vi "Frame Wall Set.vi"(8 "error in (no error)":errorcluster, 9 "Wall Stiffness (N/m)":dbl=0.2 format="%#.1f", 10 "Restrict to Frame":bool=TRUE) -> (0 "error out":errorcluster)   [LabVIEW 2023, in "Haptic Prog Interface.lvlib"]
doc: "Restricts the haptic pen xy movement to a square canvas, and coerces all xy values to be within thie canvas.\n\n<b>Restrict to Frame:</b> Accepts a boolean, where a true value enables the frame wall.\n\n<b>Wall Stiffness:</b> Accepts a double, and changes the value k in F = k x, effectively changing the hardness of the wall.."
uses:
  Haptic Prog Interface.lvlib
  Haptic-Programming-Interface/src/x64/Debug/Haptic Programming Interface.dll
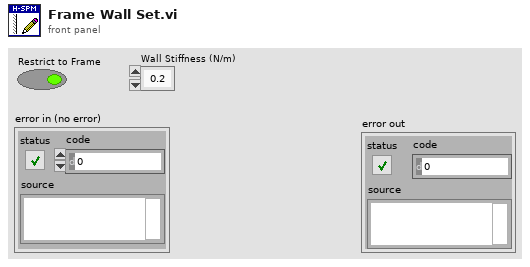
[diagram p1: front panel]
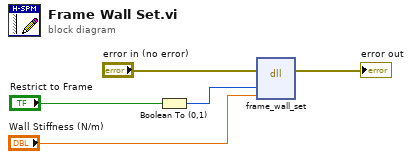
[diagram p0: block diagram]
diagram:
  n1 = Boolean To (0,1)(Boolean="Restrict to Frame") -> (0, 1=w3:i16)
  n2 = dll-call lib="C:/Users/cjwel/Documents/GitHub/Haptic-Programming-Interface/src/x64/Debug/Haptic Programming Interface.dll" fn="frame_wall_set"(error in="error in (no error)", "input"=w3, "k_wall"="Wall Stiffness (N/m)") -> (error out=→"error out":errorcluster)  [unwired: 5 in, 1 out]
